vi "motorMoveABS.vi"(4 "position":dbl, 5 "Device in":refnum<k24>) -> (2 "Device out":refnum<k24>)   [LabVIEW 2014]
doc: "André Romero - 2017\nandretec@ifsc.usp.br"
uses:
  C:/UserLab/andre/GITs/andretec/Thorlabs-Vector-Move/kinesisTec/Kinesis/Thorlabs.MotionControl.TCube.DCServoCLI.dll
  Kinesis/Thorlabs.MotionControl.TCube.DCServoCLI.dll
  motorsGlobalVar.vi
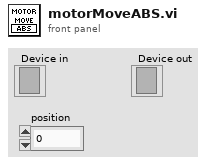
[diagram p1: front panel]
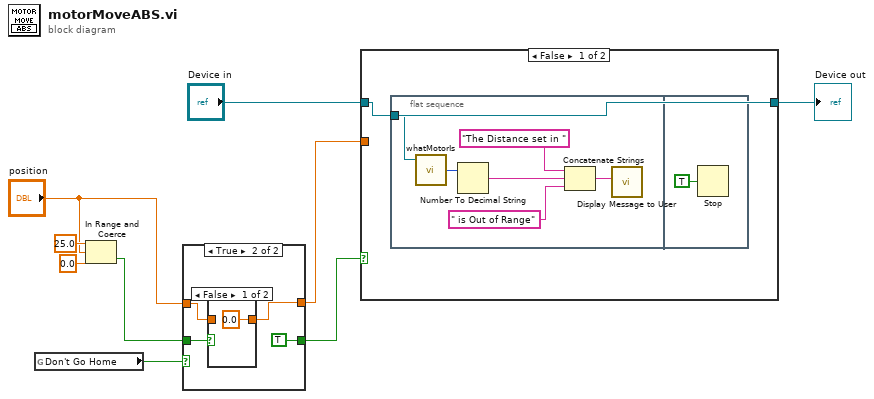
[diagram p0: block diagram]
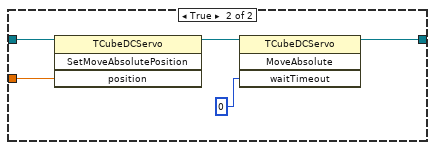
[diagram p4: hidden frame]
diagram:
  n1 = global read "motorsGlobalVar.vi" "Don't Go Home"() -> (w5:bool)
  n2 = In Range and Coerce(upper limit=25.0, x="position", lower limit=0.0) -> (In Range?=w4:bool)  [unwired: 1 out]
  n3 = case shown="True" w5 {
    tunnel: w4 -> [w11 w14]
    tunnel: [w11 TRUE] -> w3
    tunnel: "position" -> [w10 w13]
    tunnel: [w10 w12] -> w1
    frame False {
    }
    frame True {
      n4 = case shown="False" w14 {
        tunnel: w13 -> [_ w17]
        tunnel: [0.0 ("position") w17] -> w12
        frame False {
        }
        frame True {
        }
      }
    }
  }
  n5 = case shown="False" w3 {
    tunnel: "Device in" -> [w18 w30]
    tunnel: [w18 w27] -> w8
    tunnel: w1 -> [_ w29]
    frame False {
      n6 = flat-sequence {
        tunnel: w18 -> [w24]
        frame #0 {
          n7 = call "whatMotorIs.vi"("Device in"=w24) -> ("SerialNumber"=w23:u32)  [unwired: 3 in, 1 out]
          n8 = Number To Decimal String(number=w23) -> (decimal integer string=w21:string)  [unwired: 1 in]
          n9 = Concatenate Strings("The Distance set in ", w21, " is Out of Range") -> (w19:string)
          n10 = call "Display Message to User"("Message"=w19) -> ()  [unwired: 9 in, 2 out]
        }
        frame #1 {
          n11 = Stop(stop? (T)=TRUE) -> ()
        }
      }
    }
    frame True {
      n12 = invoke class="TCubeDCServo" method="SetMoveAbsolutePosition"(reference=w30, "position"=w29) -> (reference out=w28:refnum<k24>)  [unwired: 2 in, 3 out]
      n13 = invoke class="TCubeDCServo" method="MoveAbsolute"(reference=w28, "waitTimeout"=0) -> (reference out=w27:refnum<k24>)  [unwired: 2 in, 3 out]
    }
  }
  "Device out" <- w8
